vi "getFPGA.vi"(11 "ILCCommunications in":refnum<class "ILCCommunications.lvclass">) -> (2 "FPGA":refnum<class "FPGA.lvclass">, 3 "ILCCommunications out":refnum<class "ILCCommunications.lvclass">)   [LabVIEW 2016, in "ILCCommunications.lvclass"]
uses:
  ILCCommunications.lvclass
  Resources/FPGA/FPGA.lvclass
  ILCCommunications.lvclass/ILCCommunications.ctl
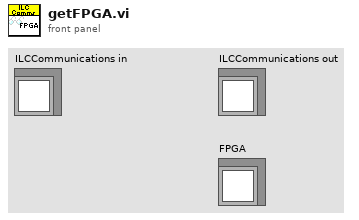
[diagram p1: front panel]
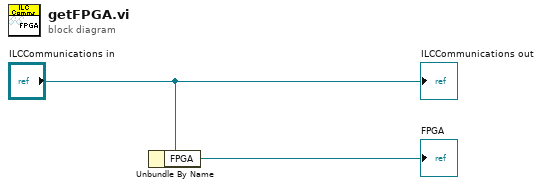
[diagram p0: block diagram]
diagram:
  n1 = Unbundle By Name("ILCCommunications in") -> ("FPGA"=→"FPGA":refnum<class "FPGA.lvclass">)
  "ILCCommunications out" <- "ILCCommunications in"
